vi "Analysator aus Definitionen löschen.vi"(10 "AnalysatorDefinitionListe":T1[](array[typedef]), 11 "Wert":T2) -> (0 "Fehler (Ausgang)":errorcluster, 3 "AnalysatorDefinitionTextListe":string[][](array[string]))   [LabVIEW 2020, in "System Einstellungen V2.lvlib"]
uses:
  System Einstellungen V2.lvlib
  Aktion FGV SystemEinstellungenV2.ctl
  Analysatoren.ctl
  AnalysatorDefinition.ctl
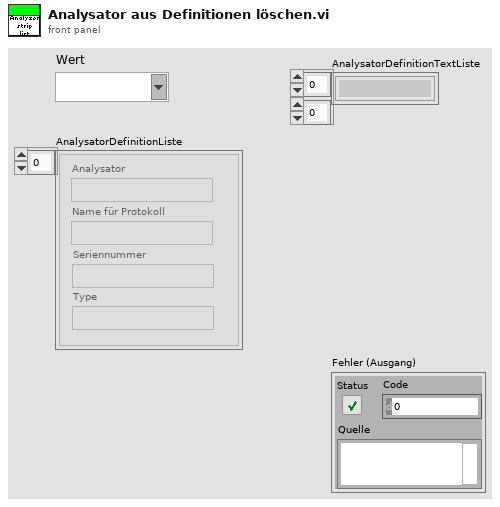
[diagram p1: front panel]
types:
  T1 = typedef "System Einstellungen V2.lvlib/AnalysatorDefinition.ctl" = cluster{"Analysator":string, "Name für Protokoll":string, "Seriennummer":string, "Type":string}
  T2 = typedef "System Einstellungen V2.lvlib/Analysatoren.ctl" = string
  T3 = typedef "System Einstellungen V2.lvlib/Aktion FGV SystemEinstellungenV2.ctl" = enum16{"lesen", "Analysatoren schreiben", "Analysator ändern", "Analysatoren löschen", "laden", "speichern", "Untertitel", "Analysatoren", "Neue Analysatoren", "Gasteiler schreiben", "Gasteiler ändern", "Gasteiler löschen", "Gasteiler", "Gasteiler exportieren", "Gasteiler importieren"}
  T4 = typedef "LVComboBoxStrsAndValuesArrayTypeDef.ctl" = cluster{"String":string, "Value":string}[]
  T5 = cluster{"AnalysatorDefinitionListe":T1[], "AnalysatorDefinitionTextListe":string[][], "Analysatoren Strings And Values[]":T4}
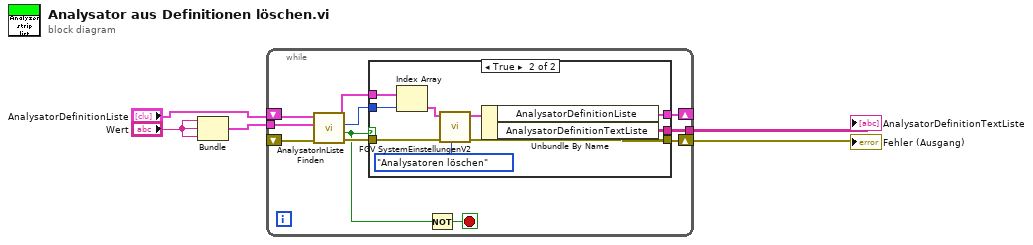
[diagram p0: block diagram]
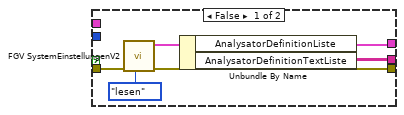
[diagram p2: hidden frame]
diagram:
  n1 = Bundle("Wert"="Wert", "Wert"="Wert", "Wert"="Wert") -> (w4:cluster{"Wert":T2, "Wert":T2, "Wert":T2})  [unwired: 1 in]
  n2 = while {
    tunnel: w4 -> [w14]
    shift-right: [w12] -> w5
    shift-left: _ -> [w11]
    shift-right: [w7] -> _
    shift-left: "AnalysatorDefinitionListe" -> [w13]
    tunnel: [w6] -> w1
    stop <- w15 stop-if-true
    n3 = call "AnalysatorInListeFinden.vi"("AnalysatorDefinition"=w14, "AnalysatorListe"=w13) -> ("gefunden"=w8:bool, "Index"=w10:i32, "AnalysatorListe out"=w9:T1[])  [unwired: 7 in]
    n4 = case shown="True" w8 {
      tunnel: [w19 w28] -> w12
      tunnel: w11 -> [w20 w27]
      tunnel: w10 -> [_ w26]
      tunnel: w9 -> [_ w25]
      tunnel: [w17 w23] -> w7
      tunnel: [w16 w22] -> w6
      frame False {
        n5 = call "FGV SystemEinstellungenV2.vi"("Aktion"=Aktion_FGV_SystemEinstellungenV2."lesen", "error in (no error)"=w20) -> ("error out"=w19:errorcluster, "Analysatoren"=w18:T5)  [unwired: 4 in, 4 out]
        n6 = Unbundle By Name(w18) -> ("AnalysatorDefinitionListe"=w17:T1[], "AnalysatorDefinitionTextListe"=w16:string[][])
      }
      frame True {
        n7 = Index Array(array=w25, index=w26) -> (element=w30:T1)
        n8 = call "FGV SystemEinstellungenV2.vi"("Aktion"=Aktion_FGV_SystemEinstellungenV2."Analysatoren löschen", "error in (no error)"=w27, "AnalysatorDefinition"=w30) -> ("error out"=w28:errorcluster, "Analysatoren"=w24:T5)  [unwired: 3 in, 4 out]
        n9 = Unbundle By Name(w24) -> ("AnalysatorDefinitionListe"=w23:T1[], "AnalysatorDefinitionTextListe"=w22:string[][])
      }
    }
    n10 = Not(x=w8) -> (.not. x?=w15:bool)
  }
  "AnalysatorDefinitionTextListe" <- w1
  "Fehler (Ausgang)" <- w5
